vi "Disconnect Standalone Wlan Card.vi"(8 "error in (no error)":errorcluster, 11 "DUT_IP":string) -> (0 "error out":errorcluster, 3 "DUT_IP out":string)   [LabVIEW 2015, in "QCA_DUT_Func.lvlib"]
doc: "DLL_QMSL_AEROFLEX void _stdcall DisconnectStandaloneWlanCard(char DUT_IP[30]);"
uses:
  QCA_DUT_Func.lvlib
  QCA_DUT_Func.dll
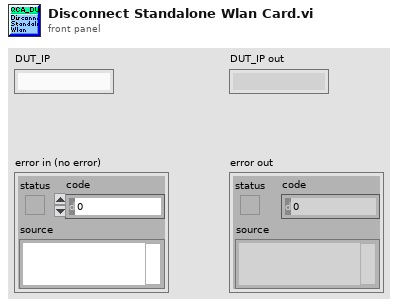
[diagram p1: front panel]
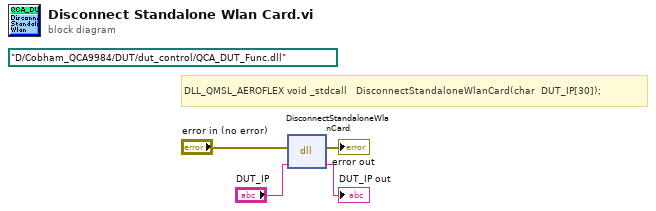
[diagram p0: block diagram]
diagram:
  (unwired) path "D:/Cobham_QCA9984/DUT/dut_control/QCA_DUT_Func.dll" ("path in")
  # "DLL_QMSL_AEROFLEX void _stdcall   DisconnectStandaloneWlanCard(char  DUT_IP[30]);"
  n1 = dll-call lib="D:/4-Up-WLAN-Test-System/DUT Control/DUT/dut_control/QCA_DUT_Func.dll" fn="DisconnectStandaloneWlanCard"(error in="error in (no error)", "DUT_IP"="DUT_IP") -> (error out=→"error out":errorcluster, "DUT_IP"=→"DUT_IP out":string)  [unwired: 3 in, 1 out]
